vi "Event Self.vi"(10 "Msg":refnum<class "Msg Strategy.lvclass">, 11 "Event Actor in":refnum<class "Event Actor.lvclass">) -> (3 "Event Actor out":refnum<class "Event Actor.lvclass">)   [LabVIEW 2021, in "jettl.lvlib" / "Event Actor.lvclass"]
uses:
  Event Actor.lvclass
  Msg Strategy/Msg Strategy/Msg Strategy.lvclass
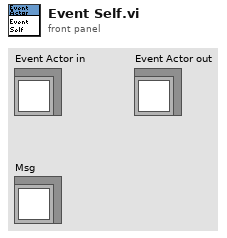
[diagram p1: front panel]
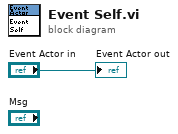
[diagram p0: block diagram]
diagram:
  "Event Actor out" <- "Event Actor in"
